vi "timer_cinetica.vi"(7 "Seconds":dbl) -> (0 "proxima":timestamp format="%<%X\n%x>T", 3 "intervalo":timestamp format="%<%X>T", 6 "ultima":timestamp format="%<%X\n%x>T")   [LabVIEW 2011]
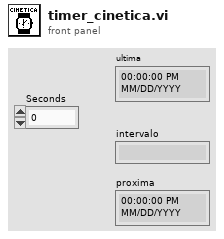
[diagram p1: front panel]
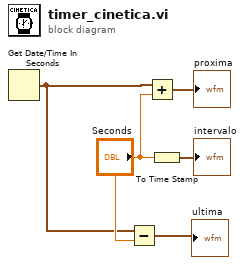
[diagram p0: block diagram]
diagram:
  n1 = Get Date/Time In Seconds() -> (seconds since 1Jan1904=w2:timestamp)
  n2 = Subtract(x=w2, y="Seconds") -> (x-y=→"ultima":timestamp)
  n3 = Add(x=w2, y="Seconds") -> (x+y=→"proxima":timestamp)
  n4 = To Time Stamp(1:"Seconds") -> (0:→"intervalo":timestamp)
